vi "Password_read.vi"(11 "error in":errorcluster) -> (1 "error out":errorcluster, 2 "Password":string, 3 "UserName":string)   [LabVIEW 2013]
uses:
  <vilib>/regexp/Match Regular Expression.xnode
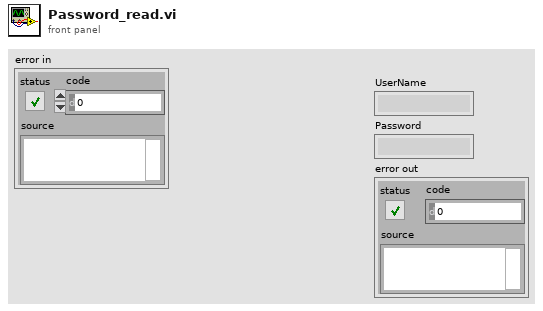
[diagram p1: front panel]
types:
  T1 = enum16{"open", "replace", "create", "open or create", "replace or create", "replace or create with confirmation"}
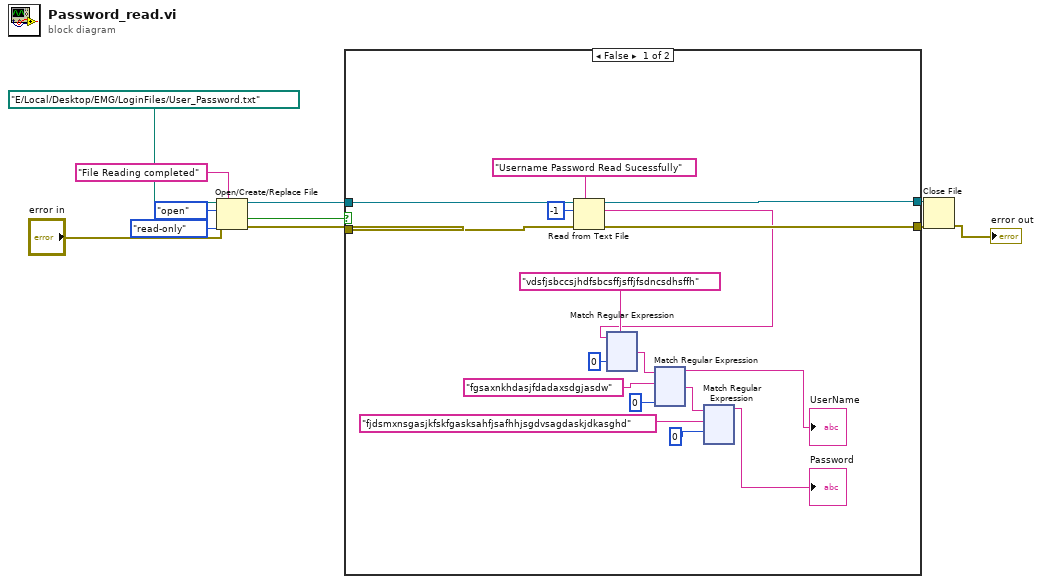
[diagram p0: block diagram]
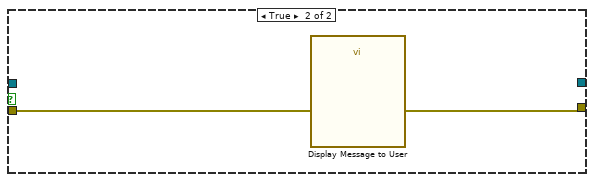
[diagram p2: hidden frame]
diagram:
  n1 = Open/Create/Replace File(file path (use dialog)=path "E:/Local/Desktop/EMG/LoginFiles/User_Password.txt", error in="error in", prompt="File Reading completed", operation (0:open)=T1."open", access (0:read/write)=enum16{"read/write", "read-only", "write-only"}."read-only") -> (refnum out=w5:refnum<file>, cancelled=w6:bool, error out=w4:errorcluster)  [unwired: 1 in]
  n2 = case shown="False" w6 {
    tunnel: w5 -> [w28 _]
    tunnel: w4 -> [w26 w371]
    tunnel: [w25 w371] -> w2
    tunnel: [w24 _] -> w3
    frame False {
      n3 = Read from Text File(prompt (Open existing file)="Username Password Read Sucessfully", file (use dialog)=w28, count=-1, error in=w26) -> (refnum out=w24:refnum<file>, text=w12:string, error out=w25:errorcluster)  [unwired: 1 out]
      n4 = xnode "Match Regular Expression"("input string"=w12, "regular expression"="vdsfjsbccsjhdfsbcsffjsffjfsdncsdhsffh", "offset (0)"=0) -> ("after match"=w16:string)  [unwired: 3 in, 4 out]
      n5 = xnode "Match Regular Expression"("input string"=w16, "regular expression"="fgsaxnkhdasjfdadaxsdgjasdw", "offset (0)"=0) -> ("before match"=→"UserName":string, "after match"=w15:string)  [unwired: 3 in, 3 out]
      n6 = xnode "Match Regular Expression"("input string"=w15, "regular expression"="fjdsmxnsgasjkfskfgasksahfjsafhhjsgdvsagdaskjdkasghd", "offset (0)"=0) -> ("before match"=→"Password":string)  [unwired: 3 in, 4 out]
    }
    frame True {
      n7 = call "Display Message to User"() -> ()  [unwired: 10 in, 2 out]
    }
  }
  n8 = Close File(refnum=w3, error in=w2) -> (error out=→"error out":errorcluster)  [unwired: 1 out]
